vi "9068_Includes.vi"   [LabVIEW 2014]
doc: "This VI's purpose is to house an instance of each runtime class that is specified within the configuration file for this target. By doing so, it ensures that all software dependencies for the configuration are present in memory before that configuration is loaded. The Standard Configuration Editor has a script that can be used to update this list of dependencies automatically.\n\nInstead of using this approach, each plug-in module could be built into a source distribution package that gets loaded into memory dynamically. This enables component-based software udpates, but requires additional configuration management effort."
uses:
  <vilib>/NI/DCAF/Engines/Standard Engine/Execution Engine/Runtime/Standard Engine Runtime.lvclass
  <vilib>/NI/DCAF/Modules/scan engine/execution/Scan Engine runtime.lvclass
  <vilib>/NI/DCAF/Modules/LED/module/execution/LED runtime.lvclass
  <vilib>/NI/DCAF/Modules/TDMS Datalogger/execution/TDMS datalogger runtime.lvclass
  <vilib>/NI/DCAF/Modules/CVT Access/execution/CVT runtime.lvclass
  <vilib>/NI/DCAF/Modules/modbus/execution/Modbus Module runtime.lvclass
  <vilib>/NI/DCAF/Modules/UDP Broadcast/execution/TEC runtime.lvclass
  <vilib>/NI/DCAF/Modules/Polynomial Scaling/module/execution/Polynomial Scale runtime.lvclass
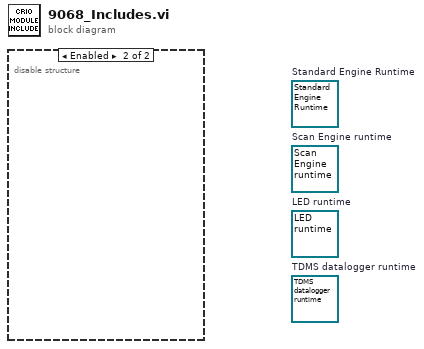
[diagram p0: block diagram]
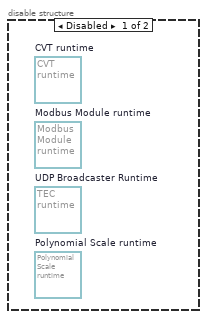
[diagram p2: hidden frame]
diagram:
  (unwired) refnum<class "TDMS datalogger runtime.lvclass"> refnum  # TDMS datalogger runtime
  (unwired) refnum<class "LED runtime.lvclass"> refnum  # LED runtime
  (unwired) refnum<class "Scan Engine runtime.lvclass"> refnum  # Scan Engine runtime
  (unwired) refnum<class "Standard Engine Runtime.lvclass"> refnum  # Standard Engine Runtime
  n1 = disable-structure shown="Enabled" {
    frame Disabled {
      (unwired) refnum<class "Polynomial Scale runtime.lvclass"> refnum  # Polynomial Scale runtime
      (unwired) refnum<class "TEC runtime.lvclass"> refnum  # UDP Broadcaster Runtime
      (unwired) refnum<class "Modbus Module runtime.lvclass"> refnum  # Modbus Module runtime
      (unwired) refnum<class "CVT runtime.lvclass"> refnum  # CVT runtime
    }
    frame Enabled {
    }
  }
